vi "Read.vi"(8 "Error in":errorcluster caption="Error in (no error)", 11 "DVR":T1) -> (0 "Error out":errorcluster, 2 "dbl":dbl, 3 "DVR(dup)":T1)   [LabVIEW 2020, in "DVR-Module.lvlib"]
uses:
  DVR-Module.lvlib
  DVR.ctl
  DataDef.ctl
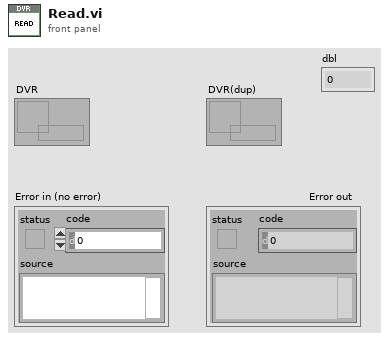
[diagram p1: front panel]
types:
  T1 = typedef "DVR-Module.lvlib/DVR.ctl" = refnum<data-value>
  T2 = typedef "DataDef.ctl" = cluster{"dbl":dbl}
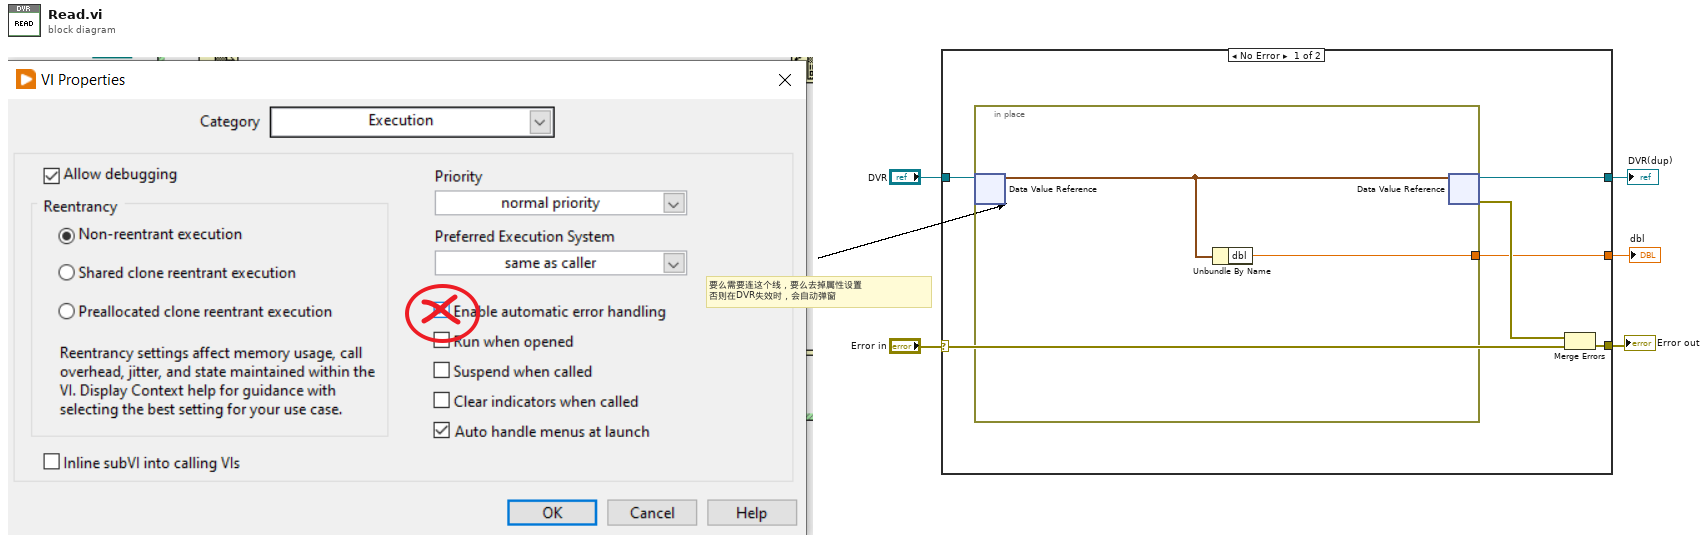
[diagram p0: block diagram]
diagram:
  # "要么需要连这个线，要么去掉属性设置\n否则在DVR失效时，会自动弹窗"
  n1 = case shown="No Error" "Error in" {
    selector: "Error in" -> [w7 w15]
    tunnel: "DVR" -> [w11 w14]
    tunnel: [w10 w14] -> w4
    tunnel: [w9 w15] -> w3
    tunnel: [w6 _] -> w1
    frame No Error {
      n2 = in-place {
        in-place-border: [w12] -> w6
        n3 = in-place-dvr #1(w11) -> (w13:T2)  [unwired: 1 out]
        n4 = Unbundle By Name(w13) -> ("dbl"=w12:dbl)
        n5 = in-place-dvr #1(w13) -> (w10:T1, w8:errorcluster)
      }
      n6 = Merge Errors(w8, w7) -> (w9:errorcluster)
    }
    frame Error {
    }
  }
  "Error out" <- w3
  "DVR(dup)" <- w4
  "dbl" <- w1
